vi "FuelAnalysis.vi"(7 "Lambda In":dbl, 8 "Counts - In":i32[][](array[numeric]), 9 "Table of Weighted Average Values - In":dbl[][](array[numeric]), 10 "RPM":dbl, 11 "Throttle Pos":dbl) -> (0 "Counts":i32[][](array[numeric]), 3 "Table of Weighted Average Values":dbl[][](array[numeric]))   [LabVIEW 2012]
panel:
  out "nearest row value":dbl
  out "nearest column value":dbl
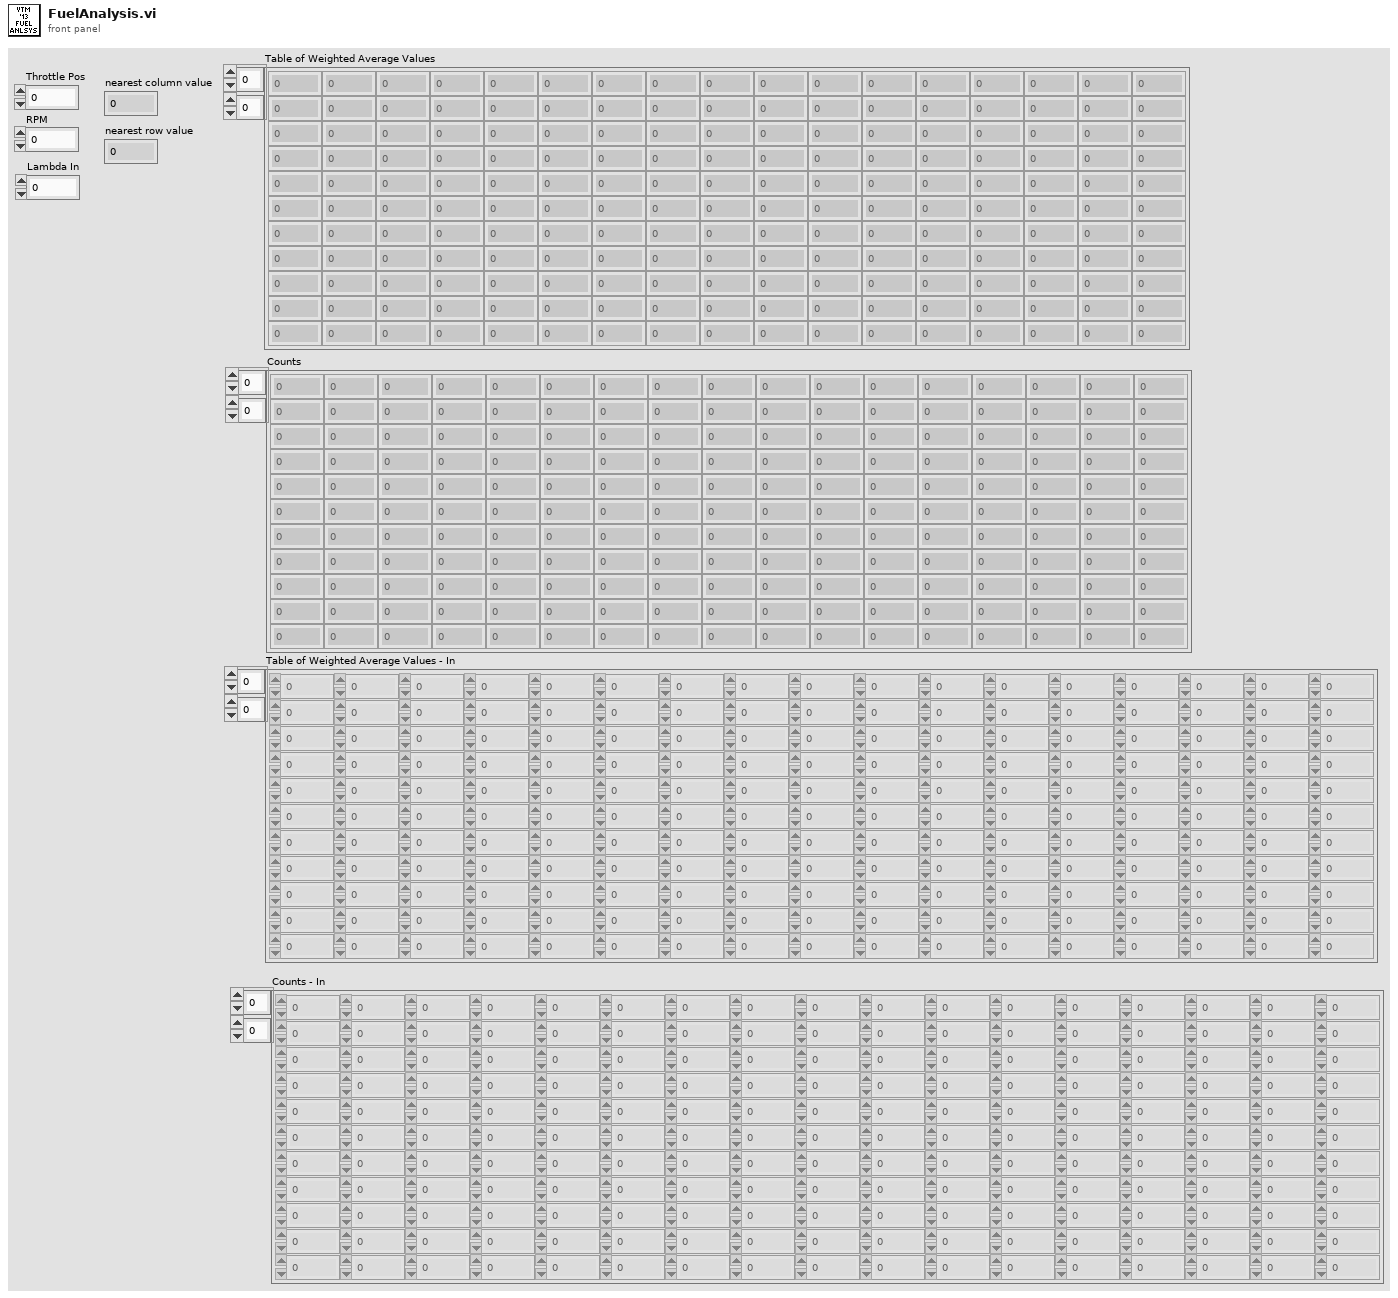
[diagram p1: front panel]
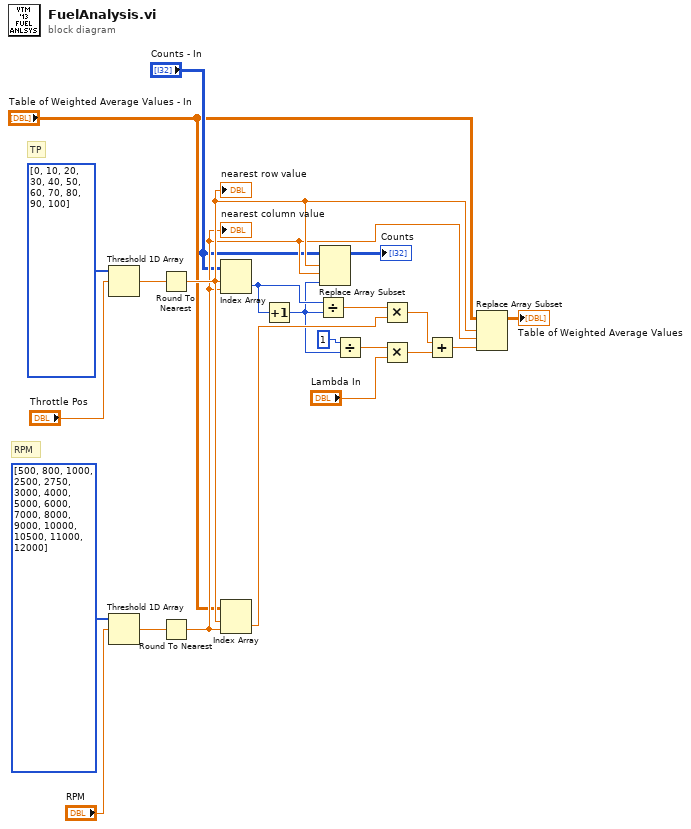
[diagram p0: block diagram]
diagram:
  # "RPM"
  # "TP"
  n1 = Threshold 1D Array(2:"Throttle Pos", 3:i32[] [0, 10, 20, 30, 40, 50, 60, 70, 80, 90, 100]) -> (0:w16:dbl)  [unwired: 1 in]
  n2 = Threshold 1D Array(2:"RPM", 3:i32[] [500, 800, 1000, 2500, 2750, 3000, 4000, 5000, 6000, 7000, 8000, 9000, 10000, 10500, 11000, 12000]) -> (0:w19:dbl)  [unwired: 1 in]
  n3 = Round To Nearest(number=w16) -> (nearest integer value=w6:dbl)
  "nearest row value" <- w6
  n4 = Round To Nearest(number=w19) -> (nearest integer value=w5:dbl)
  "nearest column value" <- w5
  n5 = Index Array(array="Counts - In", index (row)=w6, index (col)=w5) -> (element=w15:i32)
  n6 = Index Array(array="Table of Weighted Average Values - In", index (row)=w6, index (col)=w5) -> (element=w13:dbl)
  n7 = Increment(x=w15) -> (x+1=w4:i32)
  n8 = Divide(x=w15, y=w4) -> (x/y=w14:dbl)
  n9 = Replace Array Subset(array="Counts - In", new element=w4, index (row)=w6, index (col)=w5) -> (→"Counts":i32[][])
  n10 = Divide(x=1, y=w4) -> (x/y=w10:dbl)
  n11 = Multiply(x=w14, y=w13) -> (x*y=w12:dbl)
  n12 = Multiply(x=w10, y="Lambda In") -> (x*y=w8:dbl)
  n13 = Add(x=w12, y=w8) -> (x+y=w7:dbl)
  n14 = Replace Array Subset(array="Table of Weighted Average Values - In", new element=w7, index (row)=w6, index (col)=w5) -> (→"Table of Weighted Average Values":dbl[][])
